vi "Find_Rows_to_Combine.vi"(4 "Include Empty Rows?":bool, 5 "file path (dialog if empty)":path, 6 "Give Audit Channels":bool, 7 "Full Channel Names":string[](array[string]), 8 "Data":string[][](array[string]), 9 "Z Column Index":i32, 10 "Y Column Index":i32, 11 "X Column Index":i32) -> ()   [LabVIEW 2015]
uses:
  Results_plotter_Global.vi
panel:
  in  "Case Constant\n(See Context Help)":i32=1
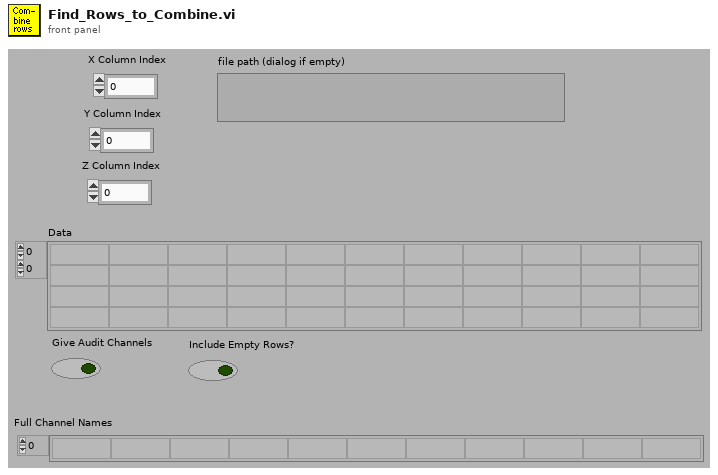
[diagram p1: front panel]
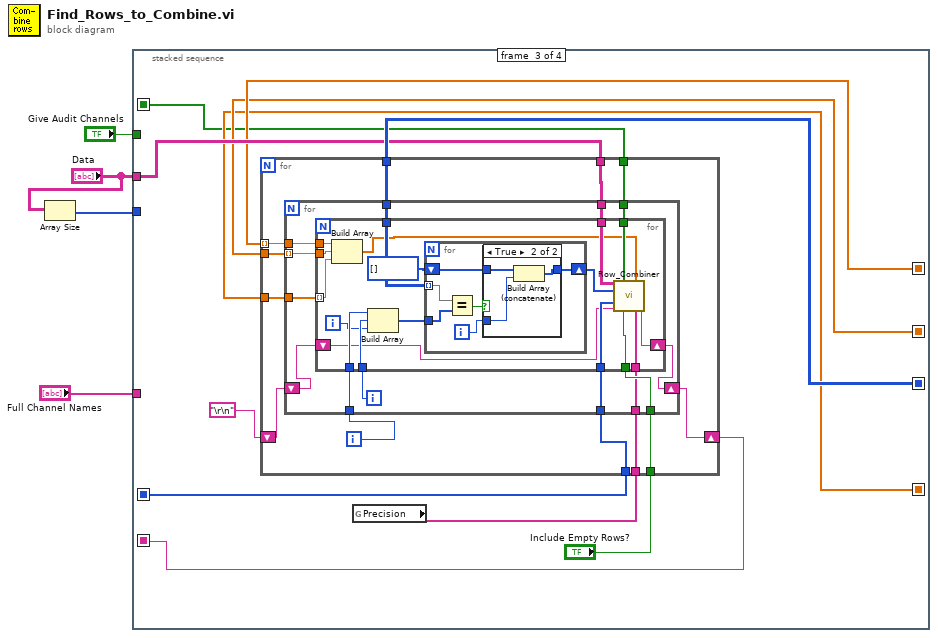
[diagram p0: block diagram]
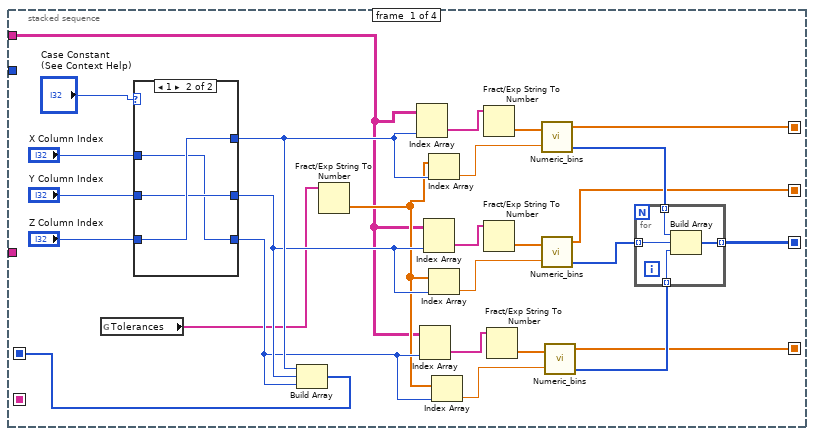
[diagram p2: hidden frame]
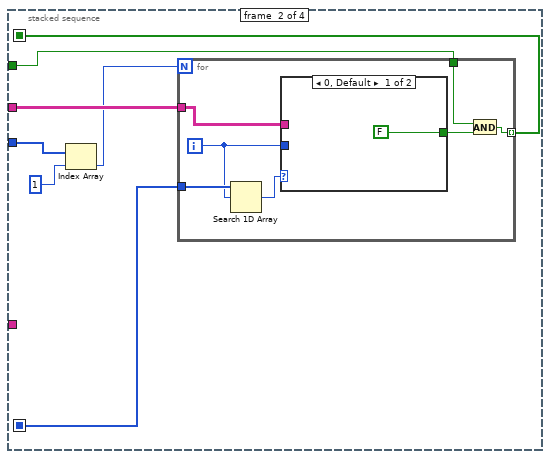
[diagram p4: hidden frame]
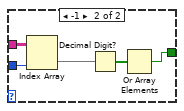
[diagram p5: hidden frame]
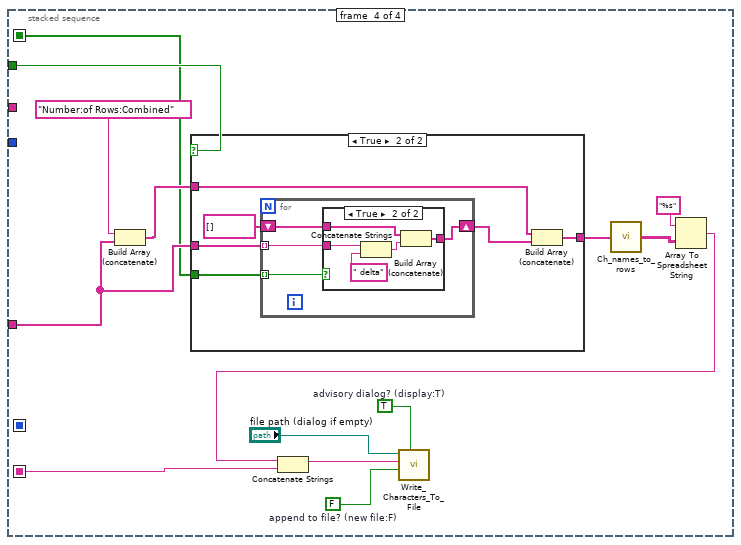
[diagram p7: hidden frame]
diagram:
  n1 = Array Size(array="Data") -> (size(s)=w1:i32[])
  n2 = stacked-sequence {
    seq-local: [w9 _ _ _] -> [_ w44 w65 _]
    seq-local: [w8 _ _ _] -> [_ _ w68 _]
    seq-local: [w7 _ _ _] -> [_ _ w67 _]
    seq-local: [w5 _ _ _] -> [_ _ w66 _]
    seq-local: [w6 _ _ _] -> [_ _ w70 _]
    seq-local: [_ _ w64 _] -> [_ _ _ w131]
    seq-local: [_ w43 _ _] -> [_ _ w63 w126]
    tunnel: "Data" -> [w10 w46 w69 _]
    tunnel: "Give Audit Channels" -> [_ w42 _ w138]
    tunnel: "Full Channel Names" -> [_ _ _ w137]
    tunnel: w1 -> [_ w47 _ _]
    frame #0 {
      n3 = global read "Results_plotter_Global.vi" "Tolerances"() -> (w11:string[])
      n4 = case shown="1" "Case Constant\n(See Context Help)" {
        tunnel: [w38 w41] -> w15
        tunnel: "X Column Index" -> [w38 w39]
        tunnel: [w37 w40] -> w14
        tunnel: "Y Column Index" -> [w37 w40]
        tunnel: [w36 w39] -> w13
        tunnel: "Z Column Index" -> [w36 w41]
        frame 0, Default {
        }
        frame 1 {
        }
      }
      n5 = Build Array(w15, w14, w13) -> (w9:i32[])
      n6 = Fract/Exp String To Number(string=w11) -> (number=w12:dbl[])  [unwired: 4 out]
      n7 = Index Array(array=w10, index (col)=w15) -> (element=w31:string[])  [unwired: 1 in]
      n8 = Index Array(array=w10, index (col)=w13) -> (element=w24:string[])  [unwired: 1 in]
      n9 = Index Array(array=w10, index (col)=w14) -> (element=w25:string[])  [unwired: 1 in]
      n10 = Index Array(array=w12, index=w15) -> (element=w29:dbl)
      n11 = Index Array(array=w12, index=w14) -> (element=w27:dbl)
      n12 = Index Array(array=w12, index=w13) -> (element=w22:dbl)
      n13 = Fract/Exp String To Number(string=w31) -> (number=w30:dbl[])  [unwired: 4 out]
      n14 = Fract/Exp String To Number(string=w25) -> (number=w26:dbl[])  [unwired: 4 out]
      n15 = Fract/Exp String To Number(string=w24) -> (number=w23:dbl[])  [unwired: 4 out]
      n16 = call "Numeric_bins.vi"("Values"=w30, "Tolerance"=w29) -> ("Bin Centres"=w8:dbl[], "Bin Index"=w21:i32[])  [unwired: 1 out]
      n17 = call "Numeric_bins.vi"("Values"=w26, "Tolerance"=w27) -> ("Bin Centres"=w7:dbl[], "Bin Index"=w20:i32[])  [unwired: 1 out]
      n18 = call "Numeric_bins.vi"("Values"=w23, "Tolerance"=w22) -> ("Bin Centres"=w5:dbl[], "Bin Index"=w19:i32[])  [unwired: 1 out]
      n19 = for {
        tunnel: w21 -> [w35] mode=indexing
        tunnel: w20 -> [w34] mode=indexing
        tunnel: w19 -> [w33] mode=indexing
        tunnel: [w32] -> w6 mode=indexing
        n20 = Build Array(w35, w34, w33) -> (w32:i32[])
      }
    }
    frame #1 {
      n21 = Index Array(array=w47, index=1) -> (element=w45:i32)
      n22 = for {
        N: w45 -> [_]
        tunnel: w46 -> [w55]
        tunnel: w44 -> [w54]
        tunnel: [w50] -> w43 mode=indexing
        tunnel: w42 -> [w49]
        i -> [w53]
        n23 = Search 1D Array(1D array=w54, element=w53) -> (index of element=w52:i32)  [unwired: 1 out]
        n24 = case shown="0, Default" w52 {
          tunnel: w55 -> [_ w61]
          tunnel: w53 -> [_ w58]
          tunnel: [FALSE w57] -> w51
          frame 0, Default {
          }
          frame -1 {
            n25 = Index Array(array=w61, index (col)=w58) -> (element=w60:string[])  [unwired: 1 in]
            n26 = Decimal Digit?(1:w60) -> (0:w59:bool[])
            n27 = Or Array Elements(Boolean array=w59) -> (logical OR=w57:bool)
          }
        }
        n28 = And(x=w49, y=w51) -> (x .and. y?=w50:bool)
      }
    }
    frame #2 {
      n29 = global read "Results_plotter_Global.vi" "Precision"() -> (w72:string[])
      n30 = for {
        tunnel: w70 -> [w84]
        tunnel: w69 -> [w82]
        tunnel: w65 -> [w81]
        shift-right: [w79] -> w64
        shift-left: "\r\n" -> [w80]
        tunnel: "Include Empty Rows?" -> [w78]
        tunnel: w68 -> [w77] mode=indexing
        tunnel: w67 -> [w76]
        tunnel: w66 -> [w75]
        tunnel: w63 -> [w74]
        tunnel: w72 -> [w73]
        i -> [w83]
        n31 = for {
          tunnel: w84 -> [w97]
          tunnel: w83 -> [w96]
          tunnel: w82 -> [w94]
          tunnel: w81 -> [w93]
          shift-right: [w91] -> w79
          shift-left: w80 -> [w92]
          tunnel: w78 -> [w90]
          tunnel: w77 -> [w89]
          tunnel: w76 -> [w88] mode=indexing
          tunnel: w75 -> [w87]
          tunnel: w74 -> [w86]
          tunnel: w73 -> [w85]
          i -> [w95]
          n32 = for {
            tunnel: w97 -> [w115]
            tunnel: w96 -> [w112]
            tunnel: w95 -> [w111]
            tunnel: w94 -> [w110]
            tunnel: w93 -> [w106]
            shift-right: [w104] -> w91
            shift-left: w92 -> [w105]
            tunnel: w90 -> [w107]
            tunnel: w89 -> [w103]
            tunnel: w88 -> [w102]
            tunnel: w87 -> [w101] mode=indexing
            tunnel: w86 -> [w100]
            tunnel: w85 -> [w98]
            i -> [w108]
            n33 = Build Array(w103, w102, w101) -> (w99:dbl[])
            n34 = Build Array(w112, w111, w108) -> (w114:i32[])
            n35 = for {
              tunnel: w115 -> [w121] mode=indexing
              tunnel: w114 -> [w120]
              shift-right: [w116] -> w109
              shift-left: i32[] [] -> [w118]
              i -> [w117]
              n36 = Equal?(x=w121, y=w120) -> (x = y?=w119:bool)
              n37 = case shown="True" w119 {
                tunnel: w118 -> [w122 w125]
                tunnel: w117 -> [_ w124]
                tunnel: [w122 w123] -> w116
                frame False {
                }
                frame True {
                  n38 = Build Array (concatenate)(w125, w124) -> (w123:i32[])
                }
              }
            }
            n39 = call "Row_Combiner.vi"("All Data"=w110, "Audit Channels"=w100, "Coordinates"=w99, "Rows to Combine"=w109, "Position Columns"=w106, "String In"=w105, "Include Empty Rows?"=w107, "Precision"=w98) -> ("String Out"=w104:string)  [unwired: 7 out]
          }
        }
      }
    }
    frame #3 {
      w127 = TRUE  # advisory dialog? (display:T)
      w128 = FALSE  # append to file? (new file:F)
      n40 = Build Array (concatenate)("Number:of Rows:Combined", w137) -> (w136:string[])
      n41 = case shown="True" w138 {
        tunnel: w137 -> [_ w146]
        tunnel: w136 -> [w140 w145]
        tunnel: [w140 w144] -> w134
        tunnel: w126 -> [_ w141]
        frame False {
        }
        frame True {
          n42 = for {
            tunnel: w146 -> [w150] mode=indexing
            shift-right: [w148] -> w142
            shift-left: string[] [] -> [w149]
            tunnel: w141 -> [w147] mode=indexing
            n43 = case shown="True" w147 {
              tunnel: w150 -> [_ w156]
              tunnel: w149 -> [w151 w153]
              tunnel: [w151 w152] -> w148
              frame False {
              }
              frame True {
                n44 = Concatenate Strings(w156, " delta" ("string")) -> (w154:string)
                n45 = Build Array (concatenate)(w153, w154) -> (w152:string[])
              }
            }
          }
          n46 = Build Array (concatenate)(w145, w142) -> (w144:string[])
        }
      }
      n47 = call "Ch_names_to_rows.vi"("Channel Names"=w134) -> ("3 Row names"=w133:string[][])
      n48 = Array To Spreadsheet String(array=w133, 3:"%s" ("format string")) -> (spreadsheet string=w132:string)  [unwired: 1 out]
      n49 = Concatenate Strings(w132, w131) -> (w130:string)
      n50 = call "Write_Characters_To_File.vi"("file path (dialog if empty)"="file path (dialog if empty)", "advisory dialog? (display:T)"=w127, "character string"=w130, "append to file? (new file:F)"=w128) -> ()  [unwired: 1 in, 4 out]
    }
  }
